vi "Write Log info.vi"(10 "Log info":string, 11 "Generic DAC Process Command in":refnum<class "Generic DAC Process Command.lvclass">) -> (3 "Generic DAC Process Command out":refnum<class "Generic DAC Process Command.lvclass">)   [LabVIEW 2019, in "DAC Process.lvlib" / "Generic DAC Process Command.lvclass"]
uses:
  Generic DAC Process Command.lvclass
  Generic DAC Process Command.lvclass/Generic DAC Process Command.ctl
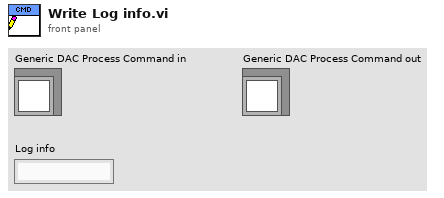
[diagram p1: front panel]
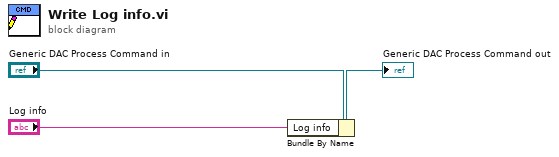
[diagram p0: block diagram]
diagram:
  n1 = Bundle By Name(cluster="Generic DAC Process Command in", "Log info"="Log info") -> (→"Generic DAC Process Command out":refnum<class "Generic DAC Process Command.lvclass">)
